vi "SetPositionUm.vi"(8 "error in (no error)":errorcluster, 9 "Positionum":dbl min=0.0 max=200.0, 10 "Stage Label":string, 11 "DemoStage in":refnum<class "DemoStage.lvclass">) -> (0 "error out":errorcluster, 3 "DemoStage out":refnum<class "DemoStage.lvclass">)   [LabVIEW 2020, in "DemoStage.lvlib" / "DemoStage.lvclass"]
uses:
  DemoStage.lvclass
  DemoStage.lvclass/DemoStage.ctl
  Hardware Abstraction Layer/Component/Stage/Stage/Stage.lvclass
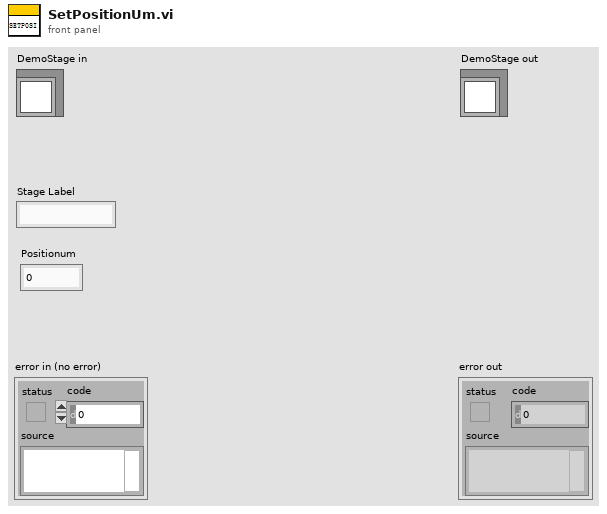
[diagram p1: front panel]
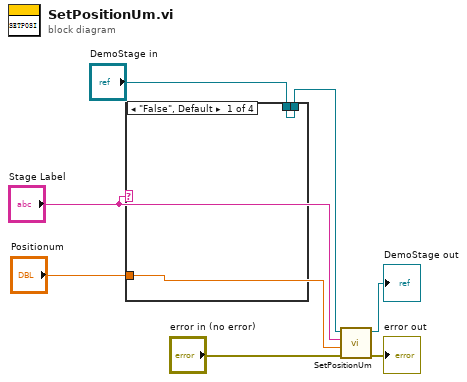
[diagram p0: block diagram]
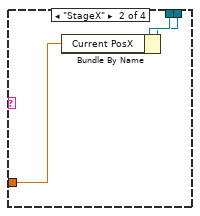
[diagram p2: hidden frame]
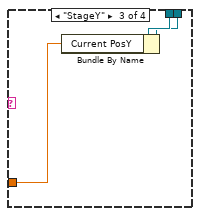
[diagram p3: hidden frame]
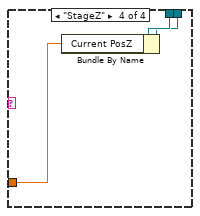
[diagram p4: hidden frame]
diagram:
  n1 = case shown="\"False\", Default" "Stage Label" {
    tunnel: "DemoStage in" -> [w8 w11 w14 w17]
    tunnel: [w8 w10 w13 w16] -> w3
    tunnel: "Positionum" -> [_ w9 w12 w15]
    frame "False", Default {
    }
    frame "StageX" {
      n2 = Bundle By Name(cluster=w11, "Current PosX"=w9) -> (w10:refnum<class "DemoStage.lvclass">)
    }
    frame "StageY" {
      n3 = Bundle By Name(cluster=w14, "Current PosY"=w12) -> (w13:refnum<class "DemoStage.lvclass">)
    }
    frame "StageZ" {
      n4 = Bundle By Name(cluster=w17, "Current PosZ"=w15) -> (w16:refnum<class "DemoStage.lvclass">)
    }
  }
  n5 = call-parent "SetPositionUm.vi"("error in (no error)"="error in (no error)", "Positionum"="Positionum", "Stage Label"="Stage Label", "Stage in"=w3) -> ("error out"=→"error out":errorcluster, "Stage out"=→"DemoStage out":refnum<class "DemoStage.lvclass">)  [unwired: 6 in]
